vi "StreamBurst with Config.vi"() -> ()   [LabVIEW 2020]
panel:
  out "StreamBurst Time [ms]":u32
  out "Combined DIO17 Count":i32
  out "Combined DIO16 Count":i32
  in  "Config Values":dbl[](array[numeric])=[10.0, 0.0, 0.0, 0.0, 0.0, 0.0, 0.0, 0.0, 7.0, 1.0, 0.0, 7.0, 1.0] format="%.2f"
  in  "Config Names":string[](array[string])=["AIN_ALL_RANGE", "STREAM_SETTLING_US", "STREAM_RESOLUTION_INDEX", "STREAM_BUFFER_SIZE_BYTES", "DIO_EF_CLOCK0_ENABLE", "DIO_EF_CLOCK1_ENABLE", "DIO_EF_CLOCK2_ENABLE", "DIO16_EF_ENABLE", "DIO16_EF_INDEX", "DIO16_EF_ENABLE", "DIO17_EF_ENABLE", "DIO17_EF_INDEX", "DIO17_EF_ENABLE"]
  in  "Number of Scans":i32=2000
  out "ConnectionType Out":i32=1
  out "DeviceType Out":i32=7
  in  "Identifier":string="LJM_idANY"
  in  "ConnectionType":string="LJM_ctANY"
  in  "DeviceType":string="LJM_dtANY"
  out "Data":dbl[][](array[numeric]) format="%.3f"
  out "Waveform Graph":dbl[][](graph)
  in  "Scan List":string[](array[string])=["AIN0", "DIO16_EF_READ_A", "STREAM_DATA_CAPTURE_16", "DIO17_EF_READ_A", "STREAM_DATA_CAPTURE_16"]
  in  "Scan Rate (Hz)":dbl=1000.0 format="%.3f"
  out "Error Message":string
  # "To remove an element, right-click\non it, select Data Operations =>\nRemove Element.\n\nTo empty an array, right-click\nnear the edge, select Data\nOperations => Empty Array.\n\nOther useful operations:  From the\nOperate menu are \"Make Current\nValues Default\" and \"Reinitialize\nTo Default\"."
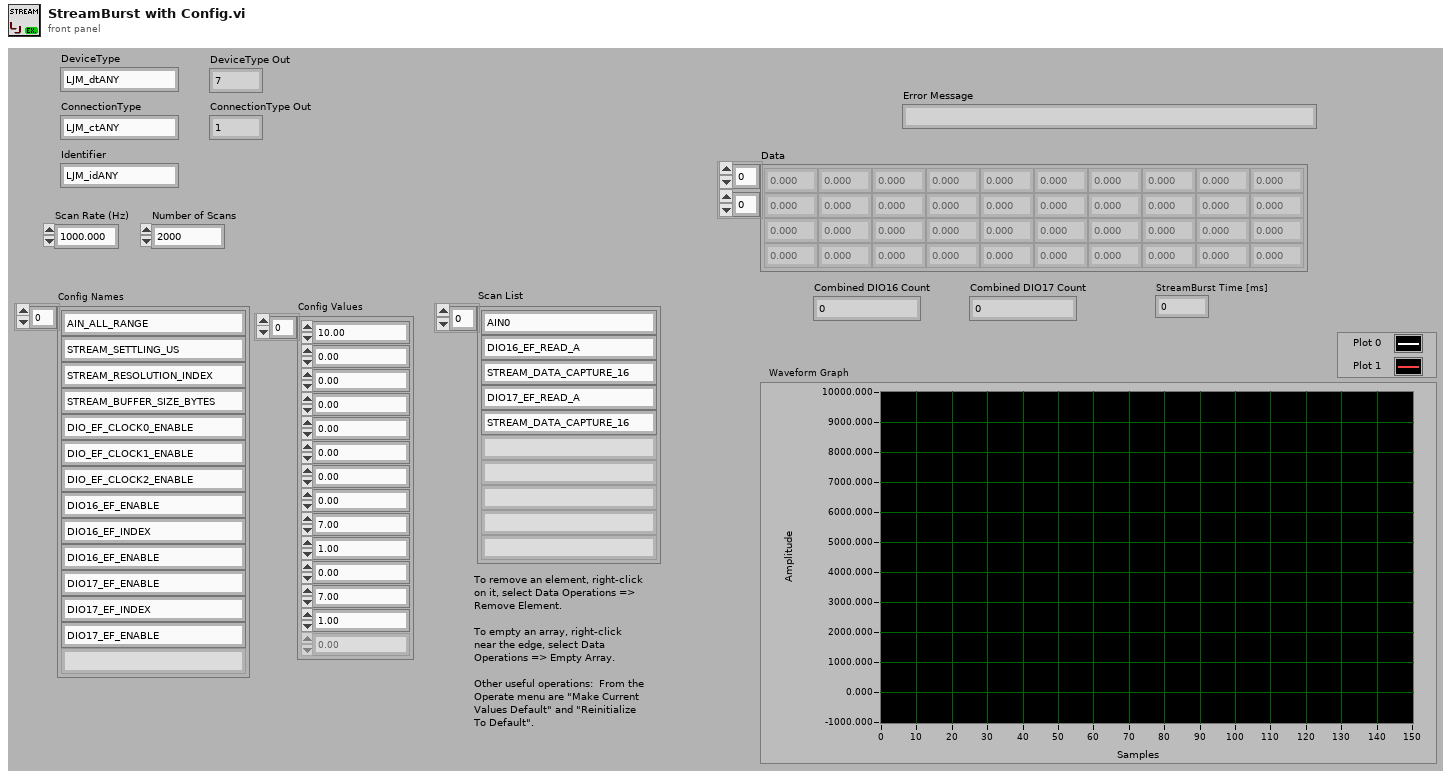
[diagram p1: front panel]
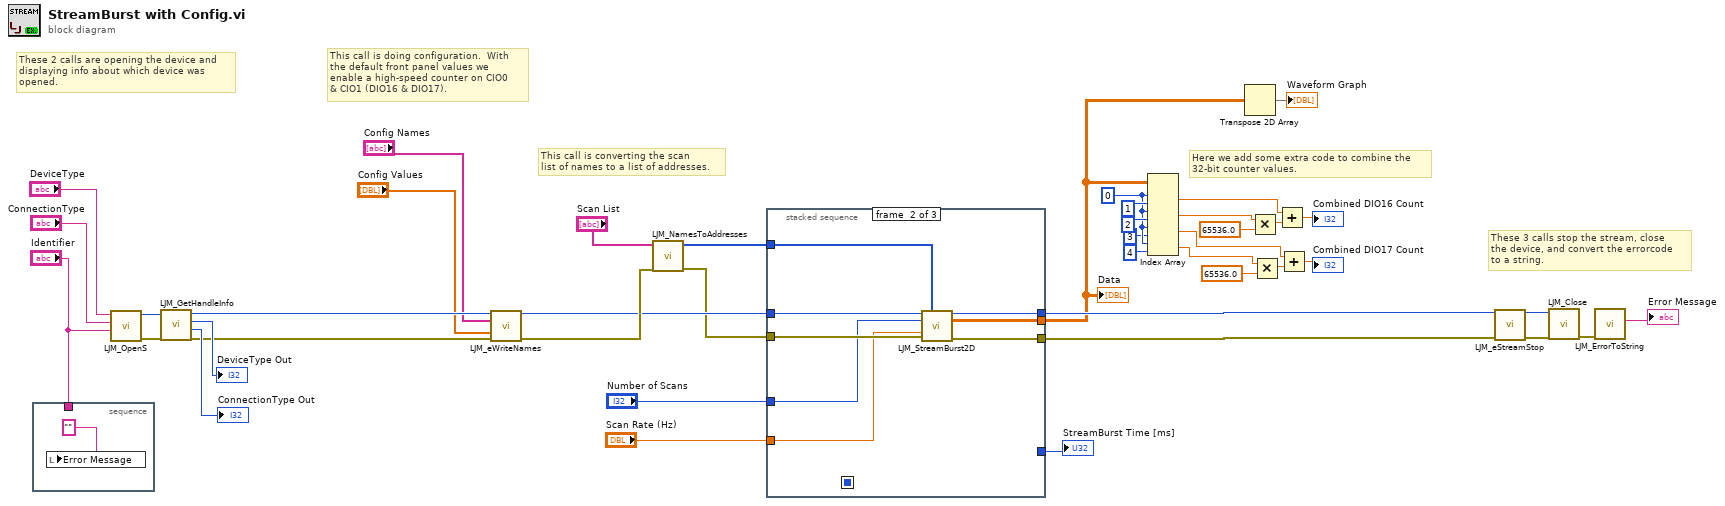
[diagram p0: block diagram]
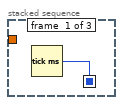
[diagram p2: hidden frame]
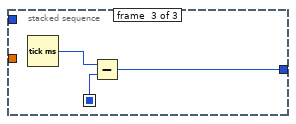
[diagram p3: hidden frame]
diagram:
  w16 = 0 ("index (row)")
  # "Here we add some extra code to combine the\n32-bit counter values."
  # "These 3 calls stop the stream, close\nthe device, and convert the errorcode\nto a string."
  # "This call is converting the scan\nlist of names to a list of addresses."
  # "This call is doing configuration.  With\nthe default front panel values we\nenable a high-speed counter on CIO0\n& CIO1 (DIO16 & DIO17)."
  # "These 2 calls are opening the device and\ndisplaying info about which device was\nopened."
  n1 = stacked-sequence {
    tunnel: "Identifier" -> [_]
    frame #0 {
      n2 = local write "Error Message"("" ("Error Message")) -> ()
    }
  }
  n3 = call "LJM_OpenS.vi"("Identifier"="Identifier", "ConnectionType"="ConnectionType", "DeviceType"="DeviceType") -> ("error out"=w36:errorcluster, "Handle"=w33:i32)  [unwired: 7 in]
  n4 = call "LJM_GetHandleInfo.vi"("error in"=w36, "Handle In"=w33) -> ("error out"=w29:errorcluster, "ConnectionType"=→"ConnectionType Out":i32, "DeviceType"=→"DeviceType Out":i32, "Handle Out"=w28:i32)  [unwired: 2 in, 4 out]
  n5 = call "LJM_eWriteNames.vi"("Handle In"=w28, "aNames"="Config Names", "aValuesIn"="Config Values", "error in"=w29) -> ("Handle Out"=w5:i32, "error out"=w27:errorcluster)  [unwired: 9 in, 1 out]
  n6 = call "LJM_NamesToAddresses.vi"("error in"=w27, "aNames"="Scan List") -> ("error out"=w4:errorcluster, "aAddresses"=w6:i32[])  [unwired: 7 in, 1 out]
  n7 = stacked-sequence {
    seq-local: [w44 _ _] -> [_ _ w54]
    tunnel: [_ w52 _] -> w42
    tunnel: [_ w51 _] -> w41
    tunnel: [_ w50 _] -> w7
    tunnel: w6 -> [_ w49 _]
    tunnel: w5 -> [_ w48 _]
    tunnel: w4 -> [_ w47 _]
    tunnel: "Number of Scans" -> [_ w46 _]
    tunnel: "Scan Rate (Hz)" -> [_ w45 _]
    tunnel: [_ _ w53] -> w1
    frame #0 {
      n8 = Tick Count (ms)() -> (millisecond timer value=w44:u32)
    }
    frame #1 {
      n9 = call "LJM_StreamBurst2D.vi"("Handle In"=w48, "aScanList"=w49, "NumScans"=w46, "ScanRate"=w45, "error in"=w47) -> ("Handle Out"=w51:i32, "aData Out"=w50:dbl[][], "error out"=w52:errorcluster)  [unwired: 8 in]
    }
    frame #2 {
      n10 = Tick Count (ms)() -> (millisecond timer value=w55:u32)
      n11 = Subtract(x=w55, y=w54) -> (x-y=w53:u32)
    }
  }
  "Data" <- w7
  "StreamBurst Time [ms]" <- w1
  n12 = Index Array(array=w7, index (row) #1=w16, index (col) #1=1 ("disabled index (col)"), index (row) #2=w16, index (col) #2=2 ("disabled index (col)"), index (row) #3=w16, index (col) #3=3 ("disabled index (col)"), index (row) #4=w16, index (col) #4=4 ("disabled index (col)")) -> (element #1=w13:dbl, element #2=w12:dbl, element #3=w11:dbl, element #4=w10:dbl)
  n13 = Transpose 2D Array(2D array=w7) -> (transposed array=→"Waveform Graph":dbl[][])
  n14 = Multiply(x=w12, y=65536.0) -> (x*y=w22:dbl)
  n15 = Multiply(x=w10, y=65536.0) -> (x*y=w19:dbl)
  n16 = Add(x=w13, y=w22) -> (x+y=→"Combined DIO16 Count":dbl)
  n17 = Add(x=w11, y=w19) -> (x+y=→"Combined DIO17 Count":dbl)
  n18 = call "LJM_eStreamStop.vi"("Handle In"=w41, "error in"=w42) -> ("Handle Out"=w39:i32, "error out"=w40:errorcluster)  [unwired: 12 in]
  n19 = call "LJM_Close.vi"("error in"=w40, "Handle"=w39) -> ("error out"=w38:errorcluster)  [unwired: 9 in]
  n20 = call "LJM_ErrorToString.vi"("error in"=w38) -> ("String"=→"Error Message":string)  [unwired: 10 in]
